vi "Iteration Check.vi"(8 "error in (no error)":errorcluster, 11 "Measurement in":refnum<class "Measurement.lvclass">) -> (0 "error out":errorcluster, 2 "Done?":bool, 3 "Measurement out":refnum<class "Measurement.lvclass">)   [LabVIEW 2017, in "Measurement Actor.lvlib" / "Measurement.lvclass"]
uses:
  Measurement.lvclass
  Measurement.lvclass/Measurement.ctl
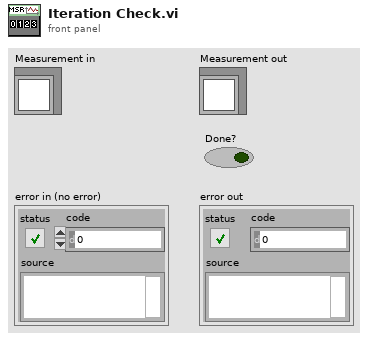
[diagram p1: front panel]
types:
  T1 = typedef "Measurement Actor.lvlib/Measurement.lvclass/Iteration count.ctl" = cluster{"Desired Iterations":i32, "Current":i32}
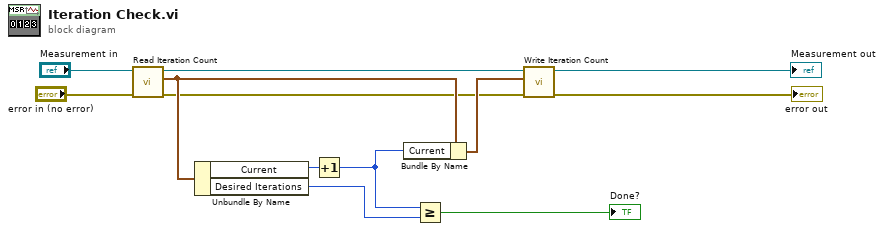
[diagram p0: block diagram]
diagram:
  n1 = call "Read Iteration Count.vi"("error in (no error)"="error in (no error)", "Measurement in"="Measurement in") -> ("error out"=w5:errorcluster, "Iteration Count"=w10:T1, "Measurement out"=w4:refnum<class "Measurement.lvclass">)  [unwired: 7 in]
  n2 = Unbundle By Name(w10) -> ("Current"=w11:i32, "Desired Iterations"=w9:i32)
  n3 = Increment(x=w11) -> (x+1=w8:i32)
  n4 = Bundle By Name(cluster=w10, "Current"=w8) -> (w7:T1)
  n5 = Greater Or Equal?(x=w8, y=w9) -> (x >= y?=→"Done?":bool)
  n6 = call "Write Iteration Count.vi"("error in (no error)"=w5, "Iteration Count"=w7, "Measurement in"=w4) -> ("error out"=→"error out":errorcluster, "Measurement out"=→"Measurement out":refnum<class "Measurement.lvclass">)  [unwired: 7 in]
